vi "Launch EMS Core.vi"(8 "error in":errorcluster, 11 "Master Controller in":refnum<class "EMS User Interface.lvclass">) -> (0 "error out":errorcluster, 3 "Master Controller out":refnum<class "EMS User Interface.lvclass">)   [LabVIEW 2018, in "EMS User Interface Actor.lvlib" / "EMS User Interface.lvclass"]
doc: "Launch SCADA. This nested actor handles all of the optimization and communication actors, so the Master Controller Core can focus on UI interaction."
uses:
  EMS User Interface.lvclass
  C:/Program Files (x86)/National Instruments/LabVIEW 2018/vi.lib/ActorFramework/Actor/Actor.lvclass
  C:/Users/Administrator/Desktop/LabVIEW EMS/EMS Generic Actor/EMS Generic/EMS Generic.lvclass
  EMS Core/EMS/EMS.lvclass
  EMS User Interface Messages/Update Microgrid State Msg/Update Microgrid State Msg.lvclass
  C:/Users/Administrator/Desktop/LabVIEW EMS/EMS Core/EMS Messages/Return Microgrid State Msg/Return Microgrid State Msg.lvclass
  EMS User Interface Messages/Update DeviceID Array Msg/Update DeviceID Array Msg.lvclass
  C:/Users/Administrator/Desktop/LabVIEW EMS/EMS Core/EMS Messages/Return DeviceID Array Msg/Return DeviceID Array Msg.lvclass
  EMS User Interface Messages/Manual Control - Connected Device Status Msg/Manual Control - Connected Device Status Msg.lvclass
  C:/Users/Administrator/Desktop/LabVIEW EMS/EMS Generic Actor/EMS Generic Messages/Return IED_Status Msg/Return IED_Status Msg.lvclass
  EMS User Interface Messages/Manual Control - Connected Device Setup Msg/Manual Control - Connected Device Setup Msg.lvclass
  C:/Users/Administrator/Desktop/LabVIEW EMS/EMS Generic Actor/EMS Generic Messages/Return DER_Info Msg/Return DER_Info Msg.lvclass
  EMS User Interface Messages/Manual Control - Connected Device Measurement Msg/Manual Control - Connected Device Measurement Msg.lvclass
  C:/Users/Administrator/Desktop/LabVIEW EMS/EMS Generic Actor/EMS Generic Messages/Return DER_Measurement Msg/Return DER_Measurement Msg.lvclass
  EMS User Interface Messages/Device State Information Update Msg/Device State Information Update Msg.lvclass
  C:/Users/Administrator/Desktop/LabVIEW EMS/EMS Generic Actor/EMS Generic Messages/Device State Information Msg/Device State Information Msg.lvclass
  EMS User Interface Messages/Current Status Update Msg/Current Status Update Msg.lvclass
  C:/Users/Administrator/Desktop/LabVIEW EMS/EMS Generic Actor/EMS Generic Messages/Return String Msg/Return String Msg.lvclass
  EMS Core/EMS/EMS.lvclass/EMS.ctl
  EMS Generic Actor/EMS Generic/EMS Generic.lvclass/EMS Generic.ctl
  EMS User Interface.lvclass/EMS User Interface.ctl
  <vilib>/ActorFramework/Actor/Actor.lvclass
  EMS Generic Actor/EMS Generic/EMS Generic.lvclass
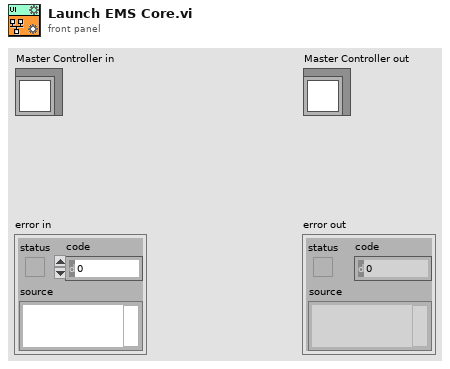
[diagram p1: front panel]
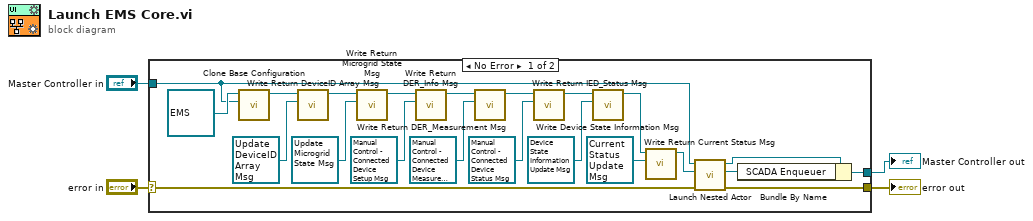
[diagram p0: block diagram]
diagram:
  n1 = case shown="No Error" "error in" {
    selector: "error in" -> [w20 w28]
    tunnel: [w23 w28] -> w3
    tunnel: [w25 w27] -> w1
    tunnel: "Master Controller in" -> [w17 w27]
    frame No Error {
      n2 = call-dynamic "Clone Base Configuration.vi"("Source Object"=w17, "Target Object in"=refnum<class "EMS.lvclass"> refnum ("SCADA Core.lvlib:SCADA.lvclass")) -> ("Target Object out"=w18:refnum<class "EMS.lvclass">)  [unwired: 9 in]
      n3 = call "Write Return DeviceID Array Msg.vi"("Return DeviceID Array Msg"=refnum<class "Update DeviceID Array Msg.lvclass"> refnum ("Master Controller Core.lvlib:Update DeviceID Array Msg.lvclass"), "SCADA in"=w18) -> ("SCADA out"=w22:refnum<class "EMS.lvclass">)  [unwired: 9 in]
      n4 = call "Write Return Microgrid State Msg.vi"("Return Microgrid State Msg"=refnum<class "Update Microgrid State Msg.lvclass"> refnum ("Master Controller Core.lvlib:Update Microgrid State Msg.lvclass"), "SCADA in"=w22) -> ("SCADA out"=w15:refnum<class "EMS.lvclass">)  [unwired: 9 in]
      n5 = call "Write Return DER_Info Msg.vi"("Return DER_Info Msg"=refnum<class "Manual Control - Connected Device Setup Msg.lvclass"> refnum ("Master Controller Core.lvlib:Manual Control - Connected Device Setup Msg.lvclass"), "EMS Generic in"=w15) -> ("EMS Generic out"=w14:refnum<class "EMS.lvclass">)  [unwired: 9 in]
      n6 = call "Write Return DER_Measurement Msg.vi"("Return DER_Measurement Msg"=refnum<class "Manual Control - Connected Device Measurement Msg.lvclass"> refnum ("Master Controller Core.lvlib:Manual Control - Connected Device Measurement Msg.lvclass"), "EMS Generic in"=w14) -> ("EMS Generic out"=w13:refnum<class "EMS.lvclass">)  [unwired: 9 in]
      n7 = call "Write Return IED_Status Msg.vi"("Return IED_Status Msg"=refnum<class "Manual Control - Connected Device Status Msg.lvclass"> refnum ("Master Controller Core.lvlib:Manual Control - Connected Device Status Msg.lvclass"), "EMS Generic in"=w13) -> ("EMS Generic out"=w9:refnum<class "EMS.lvclass">)  [unwired: 9 in]
      n8 = call "Write Device State Information Msg.vi"("Device State Information Msg"=refnum<class "Device State Information Update Msg.lvclass"> refnum ("EMS User Interface Actor.lvlib:Device State Information Update Msg.lvclass"), "EMS Generic in"=w9) -> ("EMS Generic out"=w7:refnum<class "EMS.lvclass">)  [unwired: 9 in]
      n9 = call "Write Return Current Status Msg.vi"("EMS Generic Actor.lvlib:Return String Msg.lvclass"=refnum<class "Current Status Update Msg.lvclass"> refnum ("EMS User Interface Actor.lvlib:Current Status Update Msg.lvclass"), "EMS Generic in"=w7) -> ("EMS Generic out"=w6:refnum<class "EMS.lvclass">)  [unwired: 9 in]
      n10 = call <vilib>:"Launch Nested Actor.vi"("error in (no error)"=w20, "Nested Actor"=w6, "Caller Actor in"=w17) -> ("error out"=w23:errorcluster, "Nested Actor's Enqueuer"=w24:refnum<class "Message Enqueuer.lvclass">, "Caller Actor out"=w26:refnum<class "EMS User Interface.lvclass">)  [unwired: 6 in]
      n11 = Bundle By Name(cluster=w26, "SCADA Enqueuer"=w24) -> (w25:refnum<class "EMS User Interface.lvclass">)
    }
    frame Error {
    }
  }
  "error out" <- w3
  "Master Controller out" <- w1
